vi "Write.vi"(6 "write to Cache only? (F)":bool, 7 "Qualified Name":string, 8 "error in (no error)":errorcluster, 9 "Values":variant[](array[variant]), 10 "keys":string[](array[string]), 11 "ConfigManager in":refnum<class "ConfigManager.lvclass">) -> (0 "error out":errorcluster, 2 "keys dup":string[](array[string]), 3 "ConfigManager out":refnum<class "ConfigManager.lvclass">)   [LabVIEW 2013, in "SMOConfig.lvlib" / "ConfigManager.lvclass"]
uses:
  ConfigManager.lvclass
  Cache/ConfigManager.Cache.lvclass
  ConfigManager.lvclass/ConfigManager.ctl
  Serializer/Serializer.lvclass
  Encoding/Encoding.lvclass
  Encryption/Encryption.lvclass
  <vilib>/Utility/VariantDataType/VariantType.lvlib
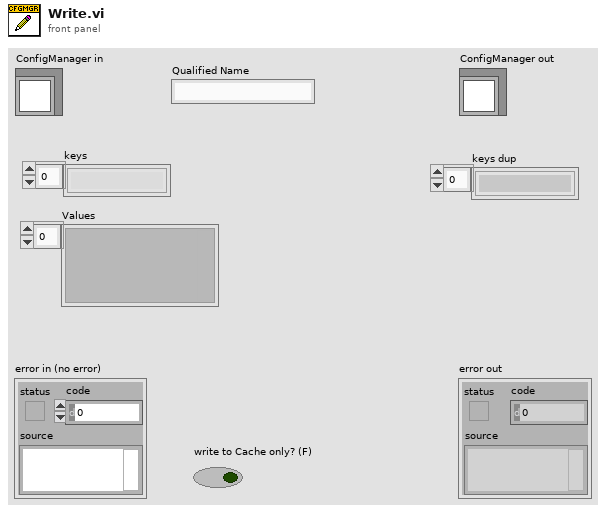
[diagram p1: front panel]
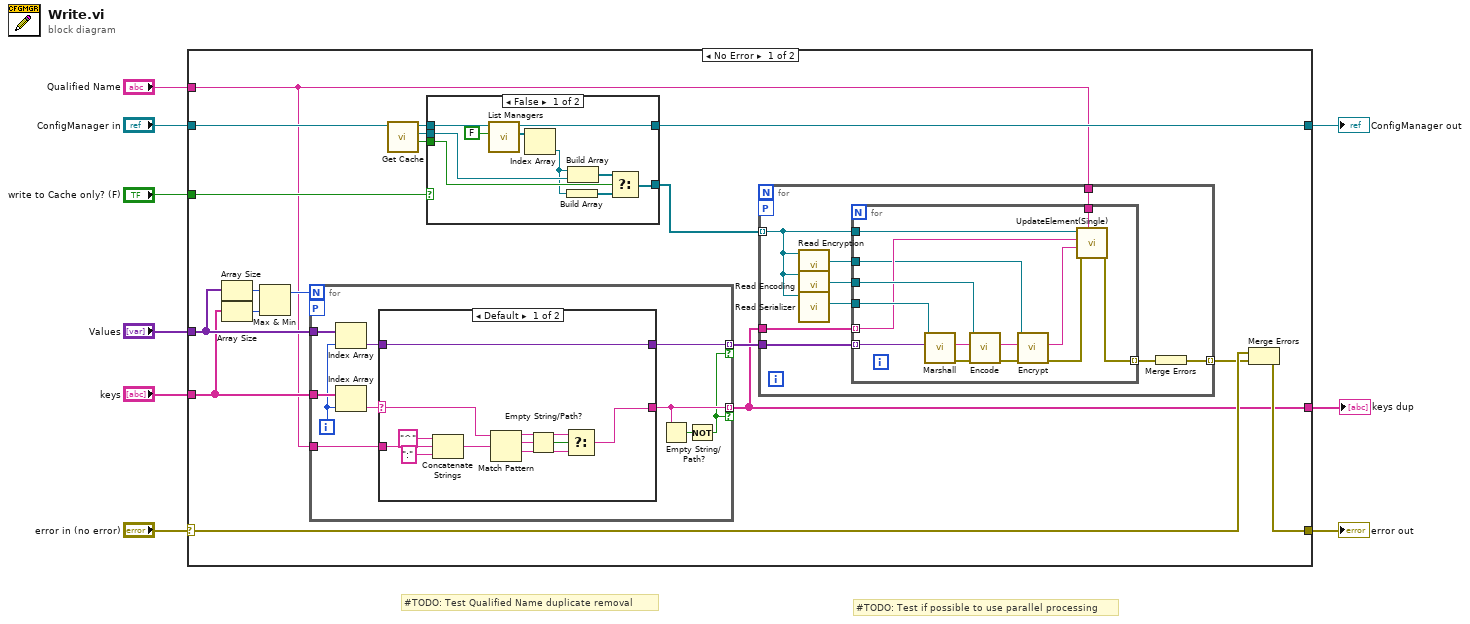
[diagram p0: block diagram]
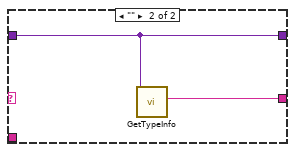
[diagram p2: hidden frame]
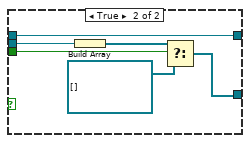
[diagram p3: hidden frame]
diagram:
  # "#TODO: Test if possible to use parallel processing"
  # "#TODO: Test Qualified Name duplicate removal"
  n1 = case shown="No Error" "error in (no error)" {
    selector: "error in (no error)" -> [w27 w90]
    tunnel: [w26 w90] -> w6
    tunnel: [w25 w89] -> w8
    tunnel: "ConfigManager in" -> [w22 w89]
    tunnel: "keys" -> [w13 w88]
    tunnel: "Values" -> [w14 _]
    tunnel: [w11 w88] -> w3
    tunnel: "Qualified Name" -> [w10 _]
    tunnel: "write to Cache only? (F)" -> [w18 _]
    frame No Error {
      n2 = Array Size(array=w14) -> (size(s)=w20:i32)
      n3 = Array Size(array=w13) -> (size(s)=w23:i32)
      n4 = Max & Min(x=w20, y=w23) -> (max(x,y)=w15:i32)  [unwired: 1 out]
      n5 = for {
        N: w15 -> [_]
        tunnel: w14 -> [w35]
        tunnel: w13 -> [w34]
        tunnel: [w32] -> w12 mode=indexing if=w29
        tunnel: [w31] -> w11 mode=indexing if=w29
        tunnel: w10 -> [w28]
        workers-P: _ -> [_]
        i -> [w33]
        n6 = Index Array(array=w35, index=w33) -> (element=w36:variant)
        n7 = Index Array(array=w34, index=w33) -> (element=w37:string)
        n8 = case shown="Default" w37 {
          selector: w37 -> [w39 _]
          tunnel: w36 -> [w48 w49]
          tunnel: [w38 w50] -> w31
          tunnel: [w48 w49] -> w32
          tunnel: w28 -> [w40 _]
          frame Default {
            n9 = Concatenate Strings("^" ("string"), w40, ":" ("string")) -> (w41:string)
            n10 = Match Pattern(string=w39, regular expression=w41) -> (before substring=w45:string, match substring=w43:string, after substring=w46:string)  [unwired: 1 in, 1 out]
            n11 = Empty String/Path?(string/path=w43) -> (empty?=w44:bool)
            n12 = Select(t=w45, s=w44, f=w46) -> (s? t:f=w38:string)
          }
          frame "" {
            n13 = call <vilib>:"GetTypeInfo.vi"("Variant"=w49) -> ("Name"=w50:string)  [unwired: 6 in, 4 out]
          }
        }
        n14 = Empty String/Path?(string/path=w31) -> (empty?=w30:bool)
        n15 = Not(x=w30) -> (.not. x?=w29:bool)
      }
      n16 = call-dynamic "Get Cache.vi"("ConfigManager in"=w22) -> ("found?"=w19:bool, "Cache"=w17:refnum<class "ConfigManager.Cache.lvclass">, "ConfigManager out"=w21:refnum<class "ConfigManager.lvclass">)  [unwired: 8 in]
      n17 = case shown="False" w18 {
        tunnel: [w75 w83] -> w16
        tunnel: [w81 w87] -> w25
        tunnel: w21 -> [w79 w87]
        tunnel: w19 -> [w76 w85]
        tunnel: w17 -> [w77 w86]
        frame False {
          n18 = call-dynamic "List Managers.vi"("Include Cache? (F)"=FALSE, "SMOConfigManager in"=w79) -> ("List"=w72:refnum<class "ConfigManager.lvclass">[], "SMOConfigManager out"=w81:refnum<class "ConfigManager.lvclass">)  [unwired: 8 in]
          n19 = Index Array(array=w72) -> (element=w73:refnum<class "ConfigManager.lvclass">)  [unwired: 1 in]
          n20 = Build Array(w73) -> (w74:refnum<class "ConfigManager.lvclass">[])
          n21 = Build Array(w73, w77) -> (w78:refnum<class "ConfigManager.lvclass">[])
          n22 = Select(t=w78, s=w76, f=w74) -> (s? t:f=w75:refnum<class "ConfigManager.lvclass">[])
        }
        frame True {
          n23 = Build Array(w86) -> (w84:refnum<class "ConfigManager.Cache.lvclass">[])
          n24 = Select(t=w84, s=w85, f=refnum<class "ConfigManager.Cache.lvclass">[] []) -> (s? t:f=w83:refnum<class "ConfigManager.Cache.lvclass">[])
        }
      }
      n25 = for {
        tunnel: [w51] -> w24 mode=indexing
        tunnel: w10 -> [w56]
        tunnel: w12 -> [w55]
        tunnel: w11 -> [w54]
        tunnel: w16 -> [w52] mode=indexing
        workers-P: _ -> [_]
        n26 = call "Read Encryption.vi"("ConfigManager in"=w52) -> ("Encryption"=w53:refnum<class "Encryption.lvclass">)  [unwired: 9 in, 1 out]
        n27 = call "Read Encoding.vi"("ConfigManager in"=w52) -> ("Encoding"=w59:refnum<class "Encoding.lvclass">)  [unwired: 9 in, 1 out]
        n28 = call "Read Serializer.vi"("ConfigManager in"=w52) -> ("Serializer"=w58:refnum<class "Serializer.lvclass">)  [unwired: 9 in, 1 out]
        n29 = for {
          tunnel: w58 -> [w66]
          tunnel: w59 -> [w70]
          tunnel: [w67] -> w57 mode=indexing
          tunnel: w55 -> [w64] mode=indexing
          tunnel: w52 -> [w69]
          tunnel: w54 -> [w63] mode=indexing
          tunnel: w56 -> [w65]
          tunnel: w53 -> [w60]
          n30 = call-dynamic "Marshall.vi"("Variant"=w64, "Serializer in"=w66) -> ("error out"=w68:errorcluster, "String"=w71:string)  [unwired: 7 in, 1 out]
          n31 = call-dynamic "Encode.vi"("String"=w71, "CfgEncoding in"=w70) -> ("Encoded String"=w62:string)  [unwired: 8 in, 1 out]
          n32 = call-dynamic "Encrypt.vi"("String"=w62, "Encryption in"=w60) -> ("Encrypted String"=w61:string)  [unwired: 8 in, 1 out]
          n33 = call-dynamic "UpdateElement(Single).vi"("Qualified Name"=w65, "error in (no error)"=w68, "Value"=w61, "Key"=w63, "SMOConfigManager in"=w69) -> ("error out"=w67:errorcluster)  [unwired: 5 in, 1 out]
        }
        n34 = Merge Errors(w57) -> (w51:errorcluster)
      }
      n35 = Merge Errors(w27, w24) -> (w26:errorcluster)
    }
    frame Error {
    }
  }
  "error out" <- w6
  "ConfigManager out" <- w8
  "keys dup" <- w3
